vi "Quit With Parameter Code.vi"   [LabVIEW 2011]
uses:
  <vilib>/Wiresmith Technology/LabVIEW CLI/CLI Class/CLI.lvclass
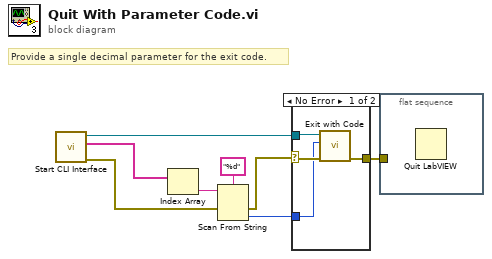
[diagram p0: block diagram]
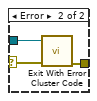
[diagram p2: hidden frame]
diagram:
  # "Provide a single decimal parameter for the exit code."
  n1 = call <vilib>:"Start CLI Interface.vi"() -> ("error out"=w4:errorcluster, "Custom Parameters"=w6:string[], "CLI out"=w8:refnum<class "CLI.lvclass">)  [unwired: 9 in]
  n2 = Index Array(array=w6) -> (element=w5:string)  [unwired: 1 in]
  n3 = Scan From String(format string="%d", input string=w5, error in=w4) -> (error out=w2:errorcluster, output 1=w1:i32)  [unwired: 2 in, 2 out]
  n4 = case shown="No Error" w2 {
    selector: w2 -> [w11 w13]
    tunnel: w8 -> [w10 w15]
    tunnel: [w12 w14] -> w7
    tunnel: w1 -> [w9 _]
    frame No Error {
      n5 = call <vilib>:"Exit with Code.vi"("error in (no error)"=w11, "Exit Code (0)"=w9, "CLI in"=w10) -> ("error out"=w12:errorcluster)  [unwired: 8 in]
    }
    frame Error {
      n6 = call <vilib>:"Exit With Error Cluster Code.vi"("error in (no error)"=w13, "CLI in"=w15) -> ("error out"=w14:errorcluster)  [unwired: 9 in]
    }
  }
  n7 = flat-sequence {
    tunnel: w7 -> [_]
    frame #0 {
      n8 = Quit LabVIEW() -> ()  [unwired: 1 in]
    }
  }
